vi "Init.vi"(8 "error in":errorcluster, 9 "Level":T1, 10 "Name":string, 11 "LokiHandler":refnum<class "LokiHandler.lvclass">) -> (0 "error out":errorcluster, 3 "LokiHandler out":refnum<class "LokiHandler.lvclass">)   [LabVIEW 2017, in "hse-logger.lvlib" / "LokiHandler.lvclass"]
doc: "Initiates a new Handler-object with a name and a log-level.\nThe handler processes LogRecords only if the level of the handler is greater or equal to the level of the LogRecord.\n\nReturns an errror \"500009 - Invalid parameter\" if ``Name`` is empty."
uses:
  LokiHandler.lvclass
  LogLevel.ctl
  Handler.lvclass
  hse-logger.lvlib
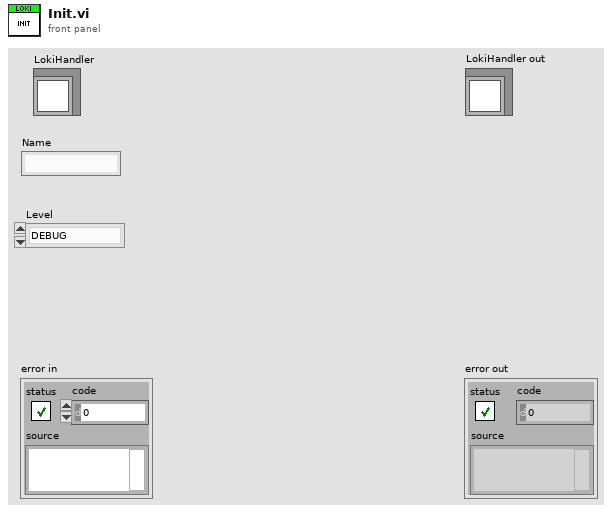
[diagram p1: front panel]
types:
  T1 = typedef "hse-logger.lvlib/LogLevel.ctl" = enum16{"DEBUG", "INFO", "WARNING", "ERROR", "CRITICAL"}
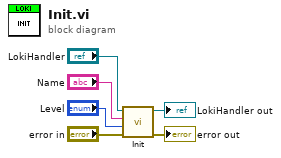
[diagram p0: block diagram]
diagram:
  n1 = call-parent "Init.vi"("error in"="error in", "Level"="Level", "Name"="Name", "Handler"="LokiHandler") -> ("error out"=→"error out":errorcluster, "Handler out"=→"LokiHandler out":refnum<class "LokiHandler.lvclass">)  [unwired: 6 in]
